vi "deinitialize.vi"(0 "HGF_Composite":refnum<class "HGF_Composite.lvclass">, 5 "error in (no error)":errorcluster) -> (19 "error out":errorcluster)   [LabVIEW 2014, in "HGF_BaseClasses.lvlib" / "HGF_Composite.lvclass"]
doc: "This is a dynamic dispatch VI. It can be overwritten by childclasses to release allocated recources."
uses:
  HGF_Composite.lvclass
  HGF_Component/HGF_Component.lvclass
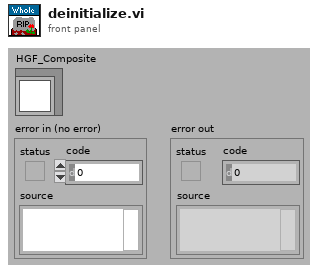
[diagram p1: front panel]
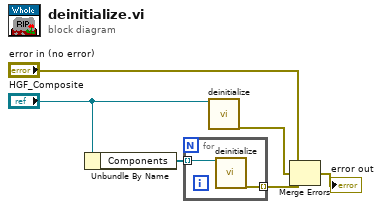
[diagram p0: block diagram]
diagram:
  n1 = Unbundle By Name("HGF_Composite") -> ("Components"=w5:refnum<class "HGF_Component.lvclass">[])
  n2 = for {
    tunnel: w5 -> [w8] mode=indexing
    tunnel: [w7] -> w4 mode=indexing
    n3 = call-dynamic "deinitialize.vi"("HGF_Factory"=w8) -> ("error out"=w7:errorcluster)  [unwired: 18 in]
  }
  n4 = call-parent "deinitialize.vi"("HGF_Factory"="HGF_Composite") -> ("error out"=w3:errorcluster)  [unwired: 1 in, 17 out]
  n5 = Merge Errors("error in (no error)", w3, w4) -> (→"error out":errorcluster)
